vi "write image timmings.vi"(8 "error in (no error)":errorcluster, 11 "Save Image in":refnum<class "Save Image.lvclass">) -> (0 "error out":errorcluster, 2 "timmings":T1, 3 "Save Image out":refnum<class "Save Image.lvclass">)   [LabVIEW 2018, in "Save Image.lvclass"]
uses:
  Save Image.lvclass
  Save Image.lvclass/Save Image.ctl
  Channel/Channel.lvclass/Channel.ctl
  Simulated_CCD_Camera/Simulated_CCD_Camera.lvclass
  Channel/Channel.lvclass
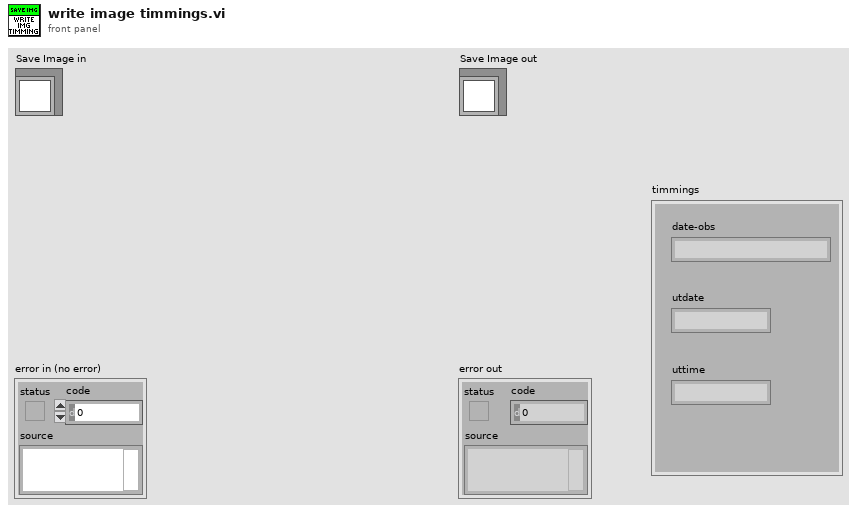
[diagram p1: front panel]
types:
  T1 = cluster{"date-obs":string, "utdate":string, "uttime":string}
  T2 = typedef "LVDateTimeRec.ctl" = cluster{"fractional second":dbl, "second":i32, "minute":i32, "hour":i32, "day of month":i32, "month":i32, "year":i32, "day of week":i32, "day of year":i32, "DST":i32}
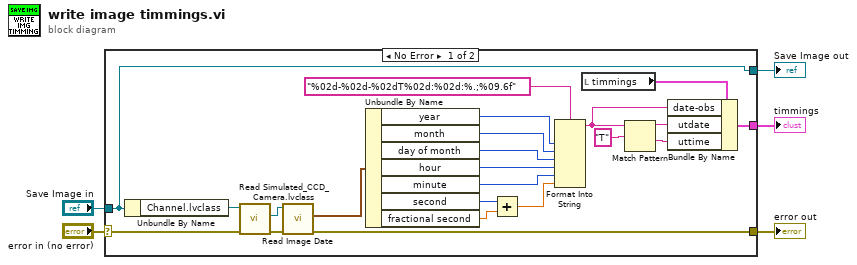
[diagram p0: block diagram]
diagram:
  n1 = case shown="No Error" "error in (no error)" {
    selector: "error in (no error)" -> [w11 w29]
    tunnel: [w9 w29] -> w4
    tunnel: [w12 w28] -> w2
    tunnel: "Save Image in" -> [w12 w28]
    tunnel: [w7 _] -> w1
    frame No Error {
      n2 = Unbundle By Name(w12) -> ("Channel.lvclass"=w13:refnum<class "Channel.lvclass">)
      n3 = call "Read Simulated_CCD_Camera.lvclass.vi"("error in (no error)"=w11, "Channel in"=w13) -> ("error out"=w10:errorcluster, "Simulated_CCD_Camera.lvclass"=w6:refnum<class "Simulated_CCD_Camera.lvclass">)  [unwired: 7 in, 1 out]
      n4 = call-dynamic "Read Image Date.vi"("error in (no error)"=w10, "Simulated_CCD_Camera in"=w6) -> ("error out"=w9:errorcluster, "SYSTEMTIME"=w19:T2)  [unwired: 7 in, 1 out]
      n5 = Unbundle By Name(w19) -> ("year"=w27:i32, "month"=w26:i32, "day of month"=w25:i32, "hour"=w24:i32, "minute"=w23:i32, "second"=w21:i32, "fractional second"=w22:dbl)
      n6 = Add(x=w21, y=w22) -> (x+y=w20:dbl)
      n7 = Format Into String(format string="%02d-%02d-%02dT%02d:%02d:%.;%09.6f", w27, w26, w25, w24, w23, w20) -> (resulting string=w18:string)  [unwired: 2 in, 1 out]
      n8 = local read "timmings"() -> (w8:T1)
      n9 = Match Pattern(string=w18, regular expression="T") -> (before substring=w16:string, after substring=w14:string)  [unwired: 1 in, 2 out]
      n10 = Bundle By Name(cluster=w8, "date-obs"=w18, "utdate"=w16, "uttime"=w14) -> (w7:T1)
    }
    frame Error {
    }
  }
  "error out" <- w4
  "Save Image out" <- w2
  "timmings" <- w1
